vi "recommendedSettings.vi"(8 "error in (no error)":errorcluster, 11 "Model in":refnum<class "Model.lvclass">) -> (0 "error out":errorcluster, 3 "Model out":refnum<class "Model.lvclass">)   [LabVIEW 2016, in "Model.lvclass"]
doc: "Publish recommended settings through SAL. Is a string with comma separated value format."
uses:
  Model.lvclass
  Model.lvclass/Model.ctl
  PubSubDataEvent/PubSubDataEvent.lvclass/PubSubDataEvent.ctl
  PubSubDataEvent/PubSubDataEvent.lvclass
  ComponentTemplateCore/ComponentModel/ComponentModel/ConfigurationFileReader/ConfigurationFileReader.lvclass
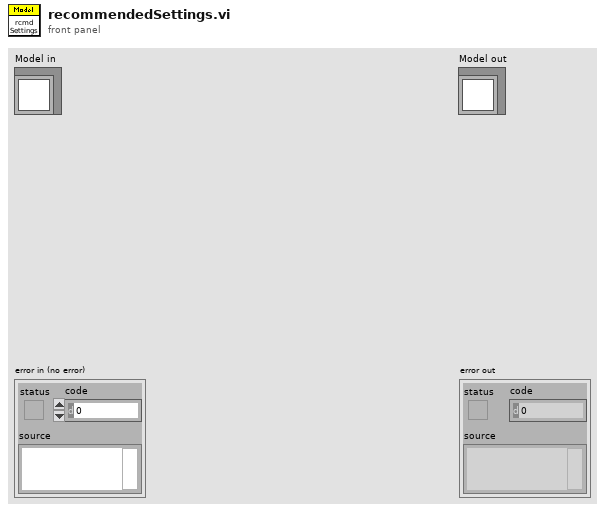
[diagram p1: front panel]
types:
  T1 = cluster{"recommendedSettingsVersion":string, "timestamp":dbl}
  T2 = typedef "EXATypedefs.lvlib/PubDataEvents.ctl" = cluster{"DetailedState":refnum<user-event>, "ErrorCode":refnum<user-event>, "Heartbeat":refnum<user-event>, "LoopTime_ms":refnum<user-event>, "LoopTimeOutOfRange":refnum<user-event>, "RejectedCommand":refnum<user-event>, "SummaryState":refnum<user-event>, "Timestamp":refnum<user-event>, "AppliedSettingsMatchStart":refnum<user-event>, "SettingsApplied":refnum<user-event>, "SettingVersions":refnum<user-event>}
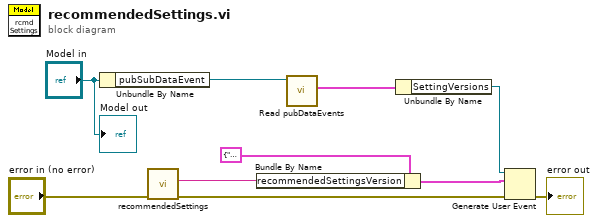
[diagram p0: block diagram]
diagram:
  n1 = Unbundle By Name("Model in") -> ("pubSubDataEvent"=w10:refnum<class "PubSubDataEvent.lvclass">)
  n2 = call "recommendedSettings.vi"("error in (no error)"="error in (no error)") -> ("error out"=w4:errorcluster, "RecommendedSettings"=w2:string)  [unwired: 8 in, 1 out]
  n3 = Bundle By Name(cluster=T1 {"recommendedSettingsVersion"="", "timestamp"=0.0} ("event data"), "recommendedSettingsVersion"=w2) -> (w1:T1)
  n4 = call "Read pubDataEvents.vi"("PubSubDataEvent in"=w10) -> ("pubDataEvents"=w8:T2)  [unwired: 9 in, 1 out]
  n5 = Unbundle By Name(w8) -> ("SettingVersions"=w7:refnum<user-event>)
  n6 = Generate User Event(user event=w7, event data cluster=w1, error in=w4) -> (error out=→"error out":errorcluster)  [unwired: 1 in, 1 out]
  "Model out" <- "Model in"
